vi "Main MSP.vi"() -> ()   [LabVIEW 2025]
uses:
  Support/Move motor.ctl
  Libraries/Control de MaP/Public/Controls/Command to motor.ctl
  Support/Stop motor.ctl
  Support/Home button.ctl
  Support/Program data--cluster.ctl
  Support/Example States.ctl
  Support/Channel configuration--cluster.ctl
  <vilib>/Instr/_visa.llb/VISA Flush IO Buffer Mask.ctl
  Libraries/Control de MaP/Public/Controls/Com Port Options.ctl
  Libraries/TDS1002 Oscilloscope/Trigger config--cluster.ctl
  Libraries/Control de MaP/Public/Write--move.vi
  <vilib>/Waveform/WDTOps.llb/WDT Get XY Value DBL.vi
  Libraries/NI DAQ/NI DAQ.lvlib
  Libraries/TDS1002 Oscilloscope/TDS1002 Oscilloscope.lvlib
  Libraries/Control de MaP/Control de MaP.lvlib
  <resource>/objmgr/daqmx.rc
panel:
  out "Driver listo":bool
  out "DAQ Mod ready":bool
  out "Osc Mod ready":bool
  in  "Connect":bool
  out "Home?":bool
  in  "Home":T1
  out "# mediciones":i32
  in  "Pasos por medición":u16=200
  out "DAQ lista":bool
  out "Osciloscopio listo":bool
  out "Status DAQ":string
  out "Osc":dbl
  in  "Detener motor":T2
  out "End":bool
  out "Posición":dbl format="%.4f"
  in  "Get position":bool
  out "Comando \nenviado":string
  in  "Motor params":T3={"Tipo"=1, "Dirección"=1, "N°. Pasos"=2000, "Frecuencia (Hz)"=255, "Tipo de paso"=2} caption="Parámetros del motor" {"Tipo de paso" items=["", "Medio paso", "Paso completo"]; "Dirección" items=["", "Izquierda", "Derecha"]; "Tipo" items=["", "Unipolar", "Bipolar"]}
  out "XY Graph":cluster{"X":dbl, "Y":dbl}[](graph)
  in  "Mover motor":T4
  in  "Driver de motor":refnum<visa-resource-name>
  in  "Osciloscopio":refnum<visa-resource-name>
  in  "DAQ":u16(ring) items=["Dev3"]
  in  "stop":bool
  # "200 pasos = 0.5mm\n1 paso = 0.0025mm\nCarrera  ~= 40mm"
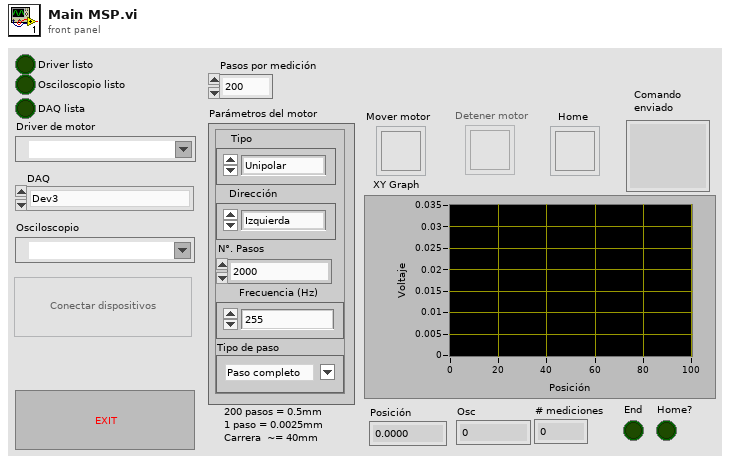
[diagram p1: front panel]
types:
  T1 = typedef "Home button.ctl" = bool
  T2 = typedef "Stop motor.ctl" = bool
  T3 = typedef "Control de MaP.lvlib/Command to motor.ctl" = cluster{"Tipo":u8, "Dirección":u8, "N°. Pasos":u16, "Frecuencia (Hz)":u8, "Tipo de paso":u8}
  T4 = typedef "Move motor.ctl" = bool
  T5 = typedef "Program data--cluster.ctl" = cluster{"Driver de motor":refnum<visa-resource-name>, "DAQ ID":i32, "TDS ID":i32, "Position":dbl, "Moving?":bool, "Pasos por medición":u16, "Motor params":T3}
  T6 = typedef "TDS1002 Oscilloscope.lvlib/Broadcast Events--cluster.ctl" = cluster{"Module Did Init":refnum<user-event>, "Status Updated":refnum<user-event>, "Error Reported":refnum<user-event>, "Module Did Stop":refnum<user-event>, "Update Module Execution Status":refnum<user-event>, "Helper Loop Status Updated":refnum<user-event>, "Device connected":refnum<user-event>, "Device disconnected":refnum<user-event>, "Data acquired":refnum<user-event>, "Configuration applied":refnum<user-event>}
  T7 = typedef "NI DAQ.lvlib/Broadcast Events--cluster.ctl" = cluster{"Module Did Init":refnum<user-event>, "Status Updated":refnum<user-event>, "Error Reported":refnum<user-event>, "Module Did Stop":refnum<user-event>, "Update Module Execution Status":refnum<user-event>, "Digital data acquired":refnum<user-event>, "Device connected":refnum<user-event>, "Connection failed":refnum<user-event>, "Analog data acquired":refnum<user-event>, "Tasks started":refnum<user-event>}
  T8 = typedef "Example States.ctl" = enum16{"Wait", "Validate connection", "Validate modules", "Connect", "Initialize", "Stop motor", "Error", "Exit"}
  T9 = enum8{"Enabled", "Disabled", "Disabled and Grayed Out"}
  T10 = typedef "TDS1002 Oscilloscope.lvlib/Trigger config--cluster.ctl" = cluster{"Trigger Source":i32, "Trigger Mode":i32, "Trigger Slope":i32, "Trigger Coupling":i32, "Trigger Level":dbl}
  T11 = enum16{"All", "DO task", "DI task", "AO task", "AI task"}
  T12 = typedef "TDS1002 Oscilloscope.lvlib/Channel configuration--cluster.ctl" = cluster{"Acquisition Type":i32, "Averaged Waveforms":i32, "Channel":i32, "Probe Attenuation":i32, "Timebase":dbl}
  T13 = typedef "VISA Flush IO Buffer Mask.ctl" = u16
  T14 = typedef "Control de MaP.lvlib/Com Port Options.ctl" = cluster{"baud rate (9600)":u32, "data bits (8)":u16, "parity (0:none)":enum16{"None", "Odd", "Even", "Mark", "Space"}}
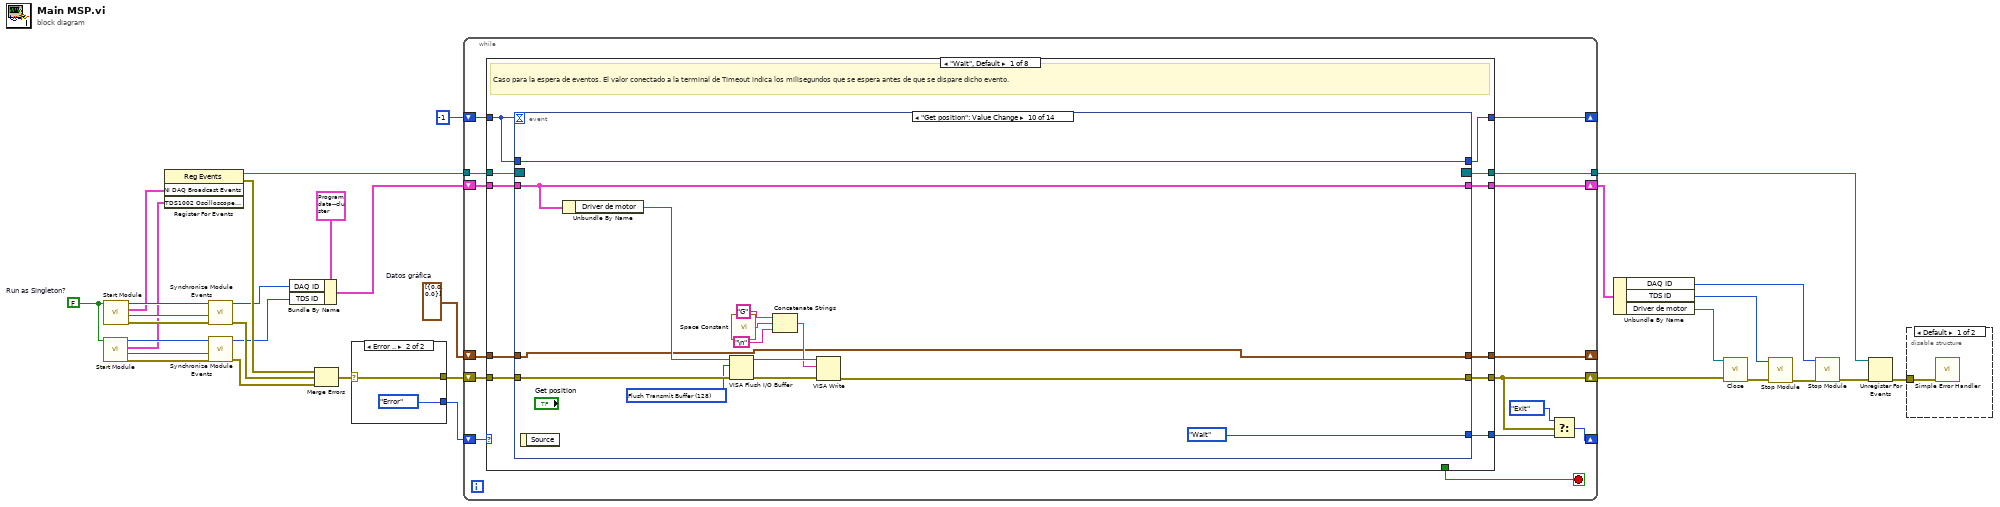
[diagram p0: block diagram]
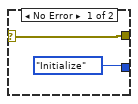
[diagram p2: hidden frame]
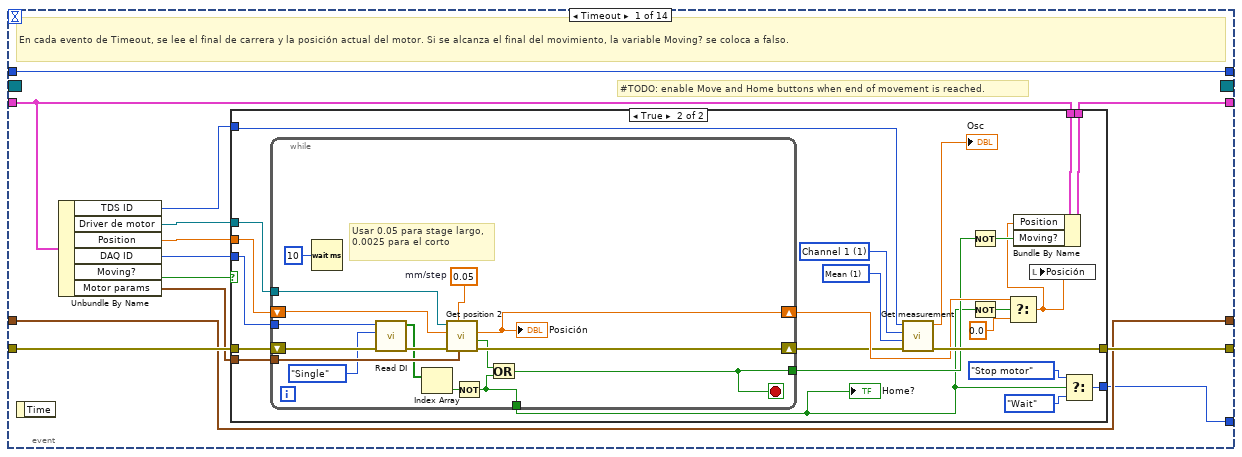
[diagram p3: hidden frame]
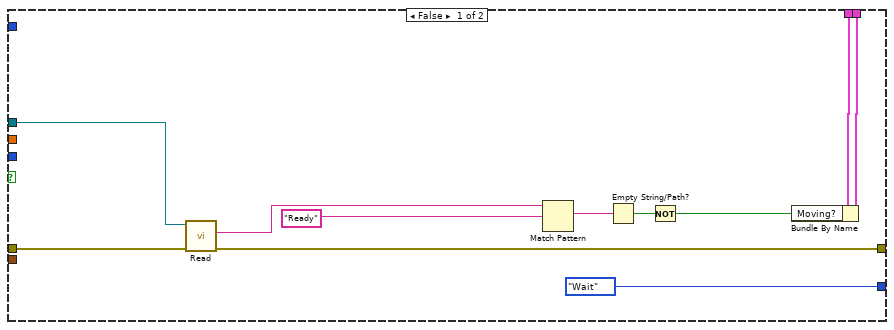
[diagram p4: hidden frame]
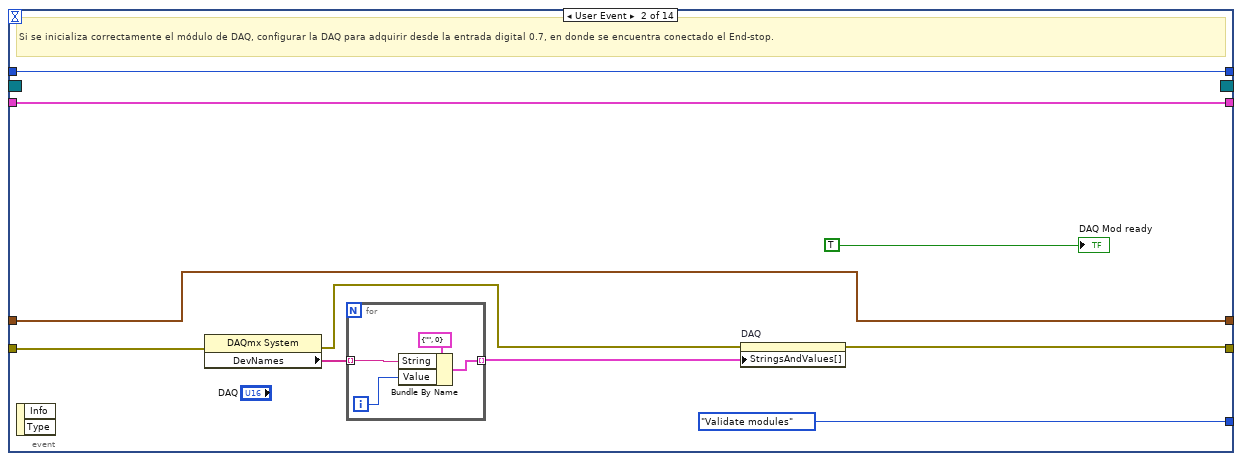
[diagram p5: hidden frame]
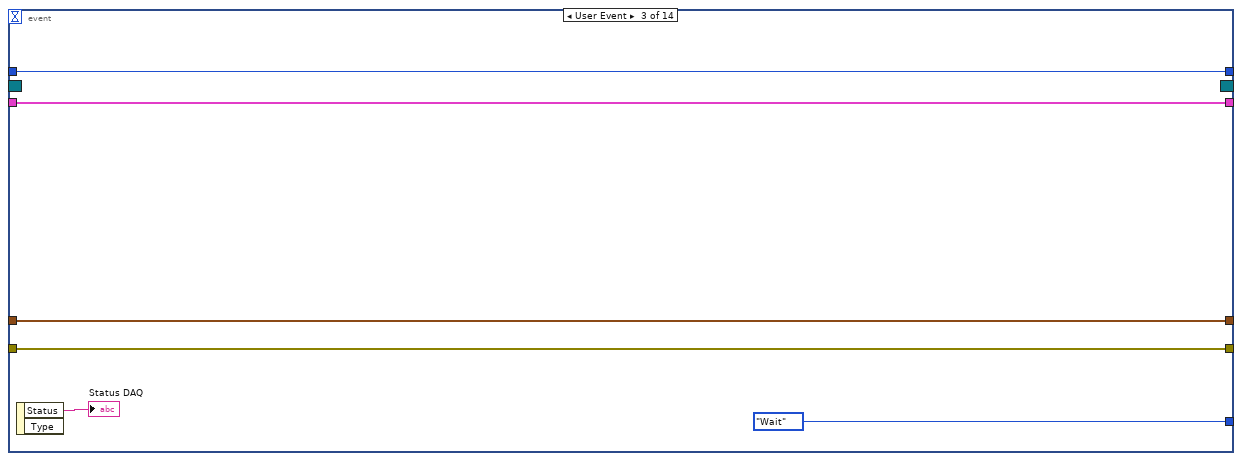
[diagram p6: hidden frame]
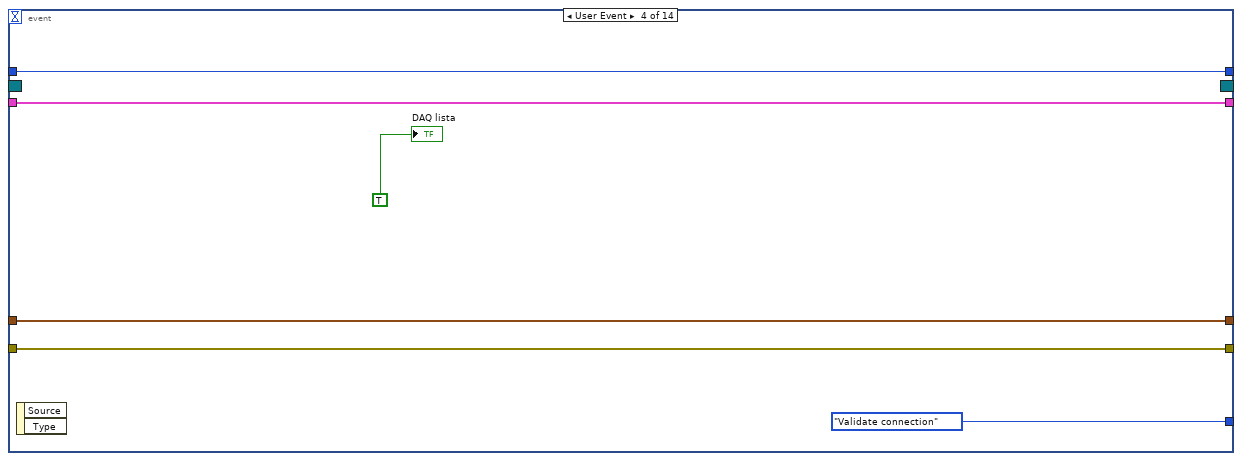
[diagram p7: hidden frame]
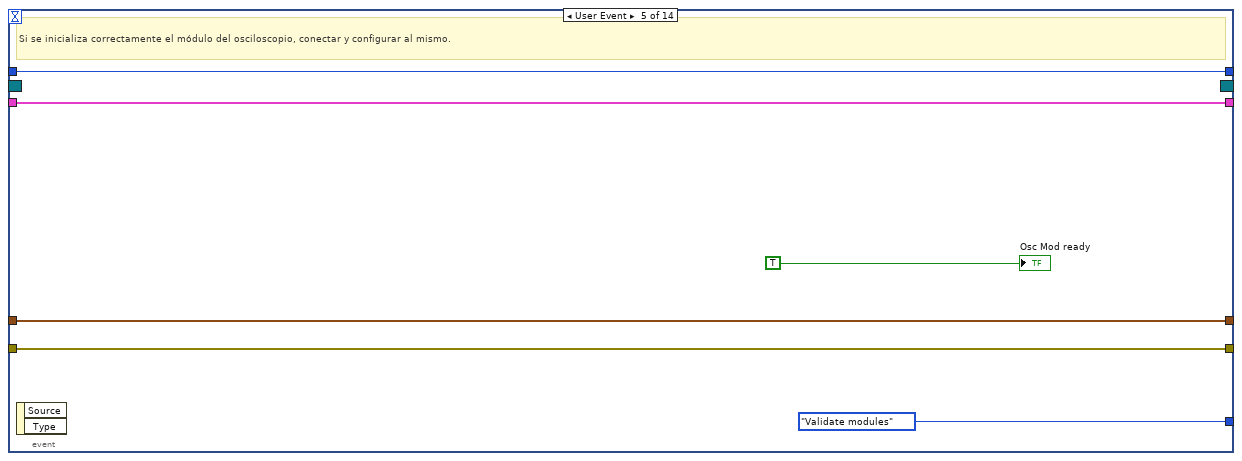
[diagram p8: hidden frame]
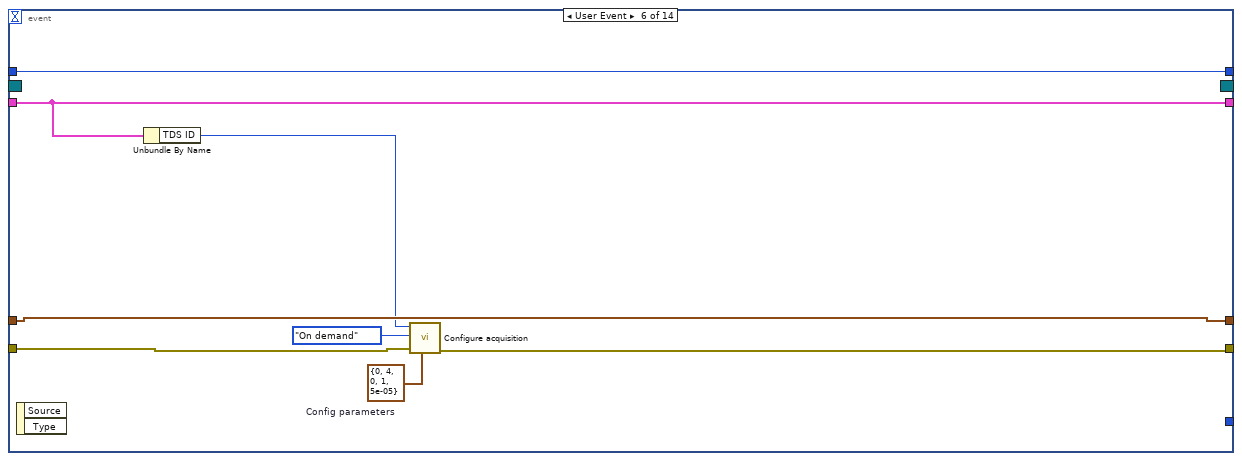
[diagram p9: hidden frame]
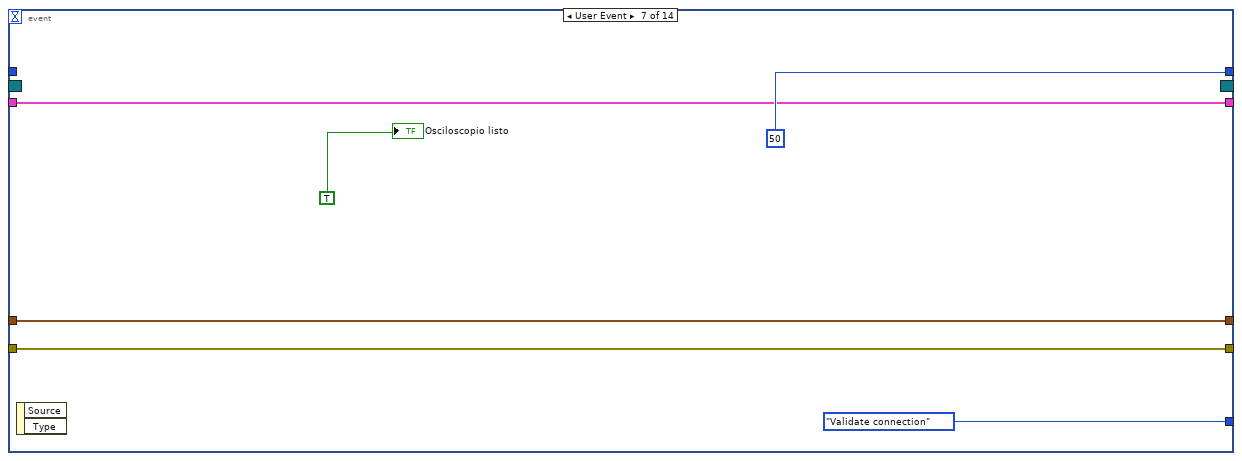
[diagram p10: hidden frame]
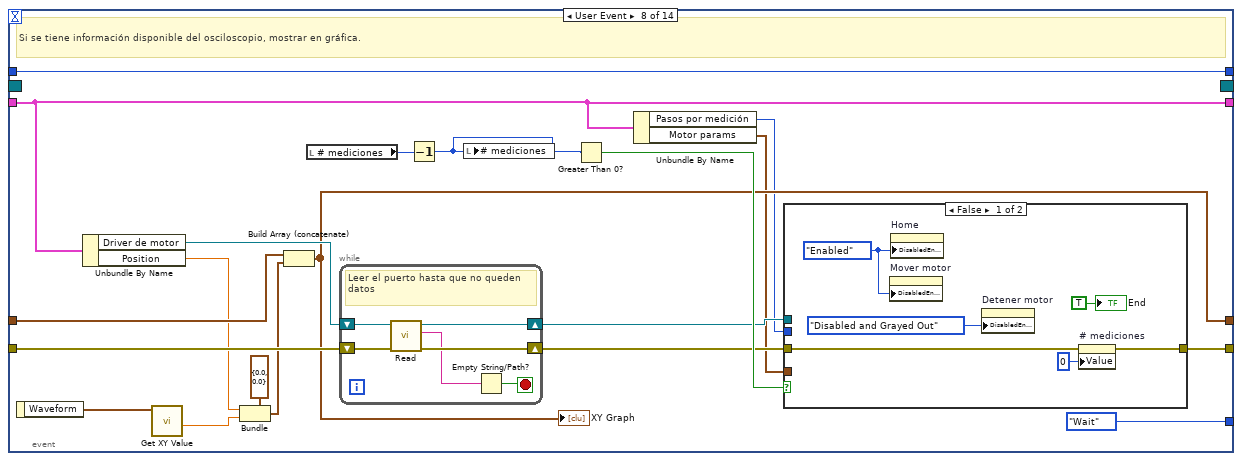
[diagram p11: hidden frame]
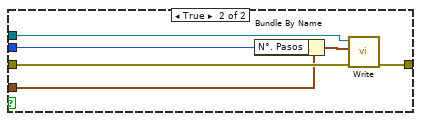
[diagram p12: hidden frame]
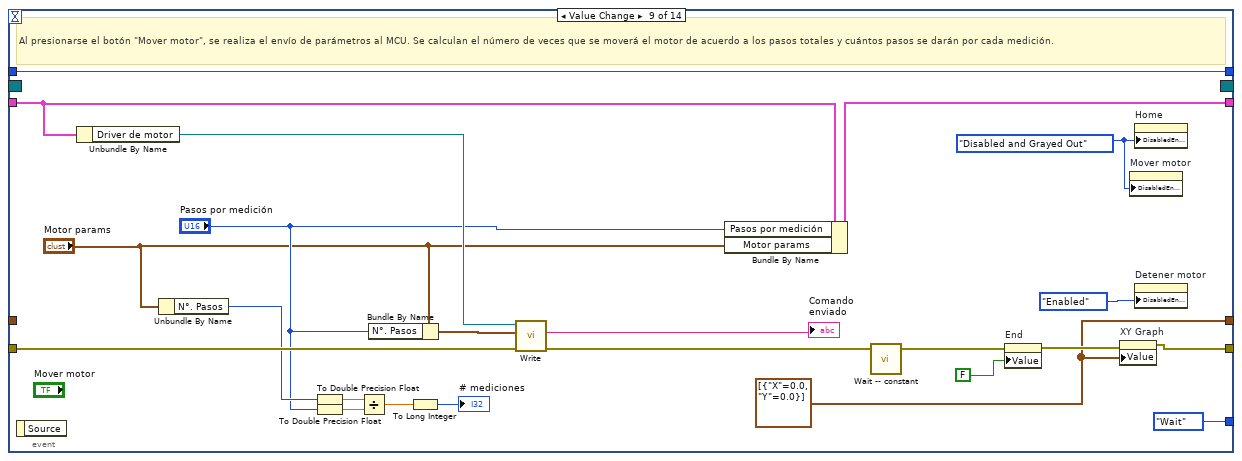
[diagram p13: hidden frame]
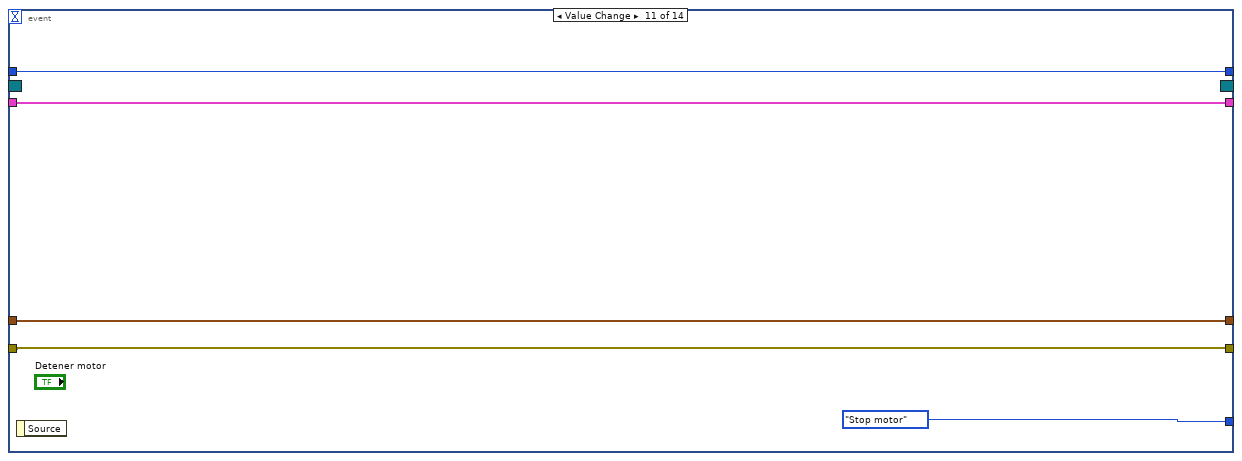
[diagram p14: hidden frame]
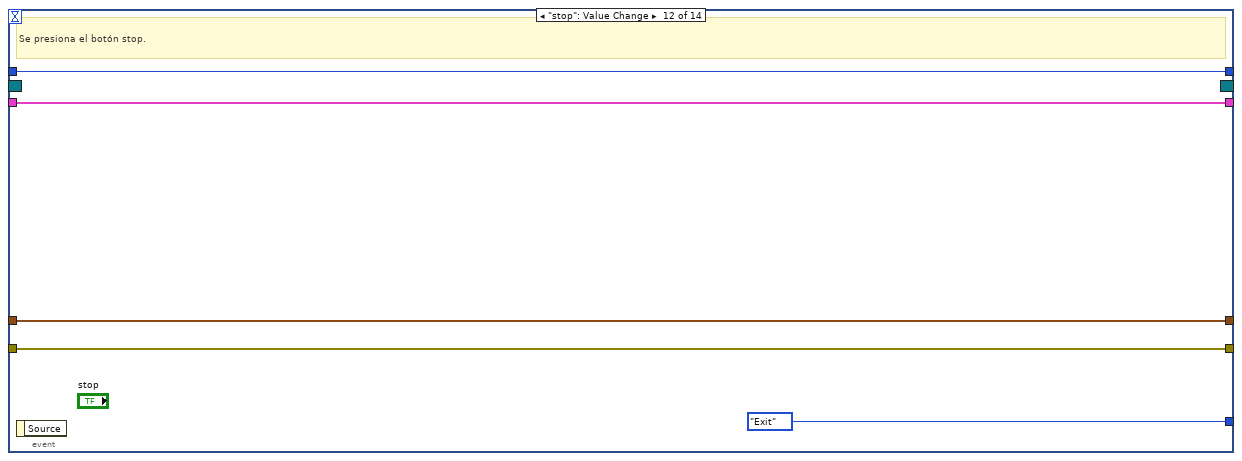
[diagram p15: hidden frame]
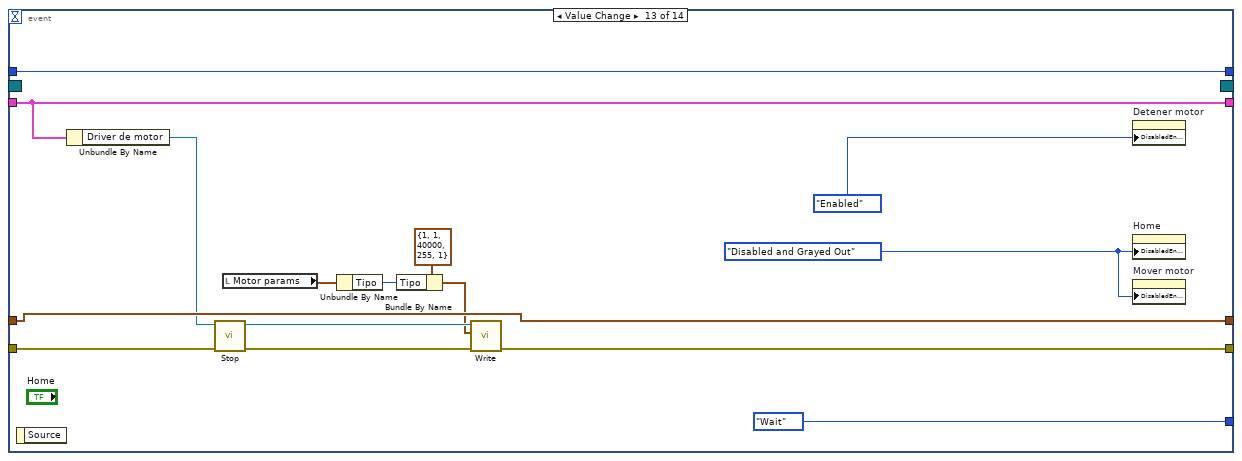
[diagram p16: hidden frame]
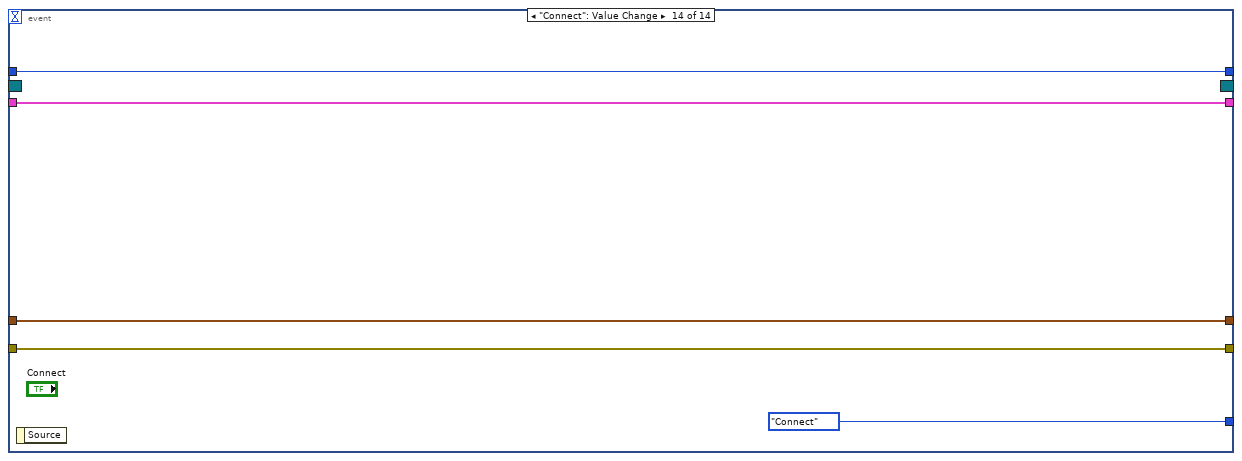
[diagram p17: hidden frame]
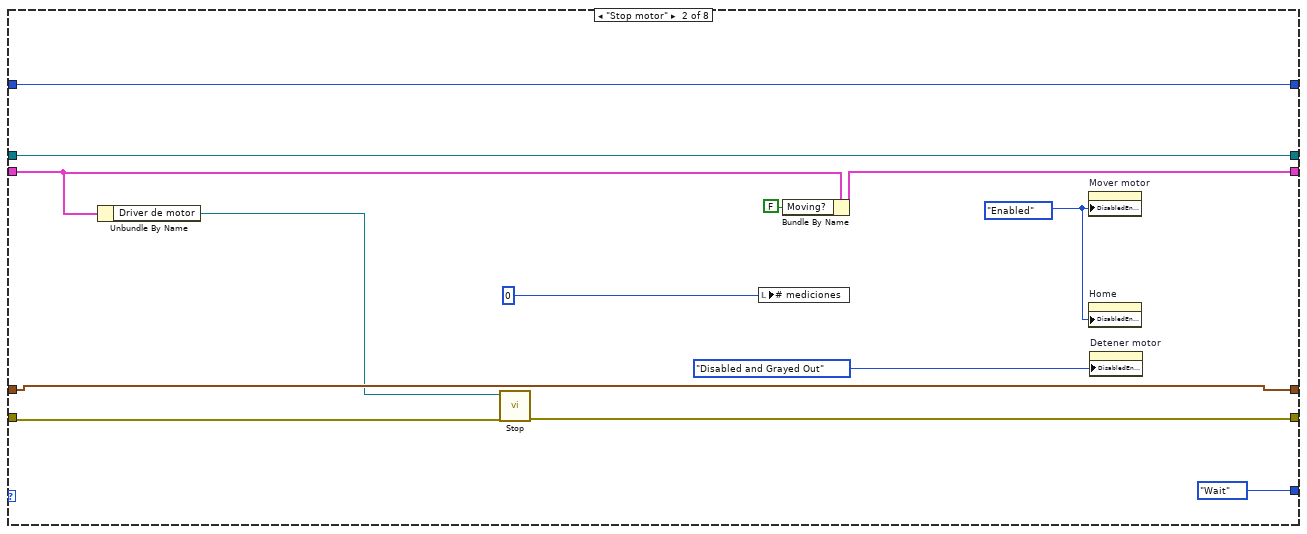
[diagram p18: hidden frame]
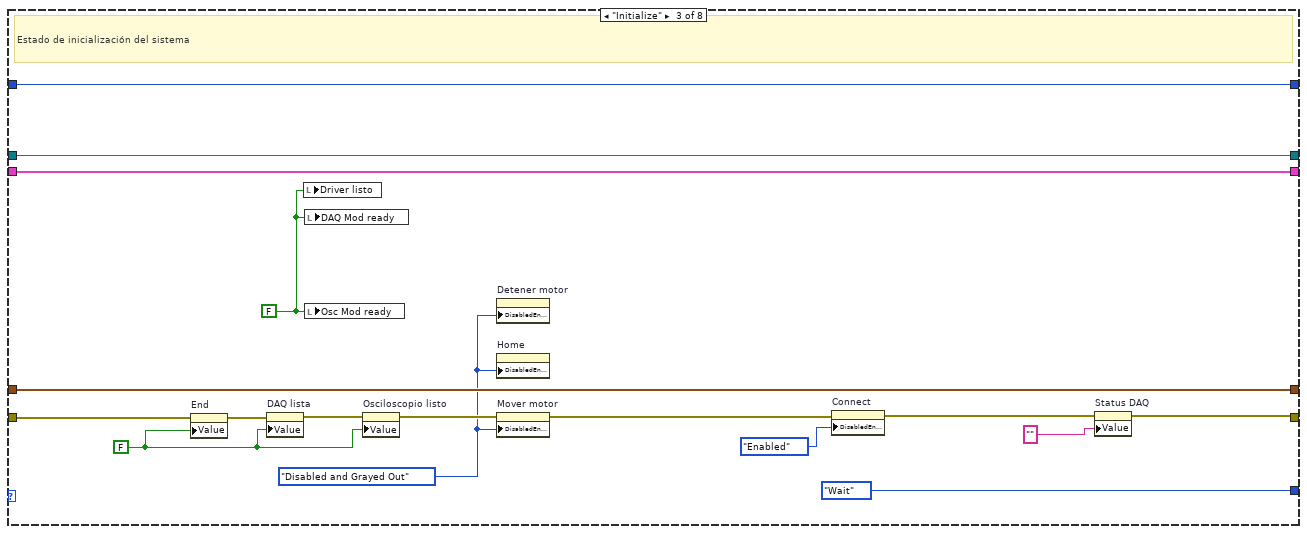
[diagram p19: hidden frame]
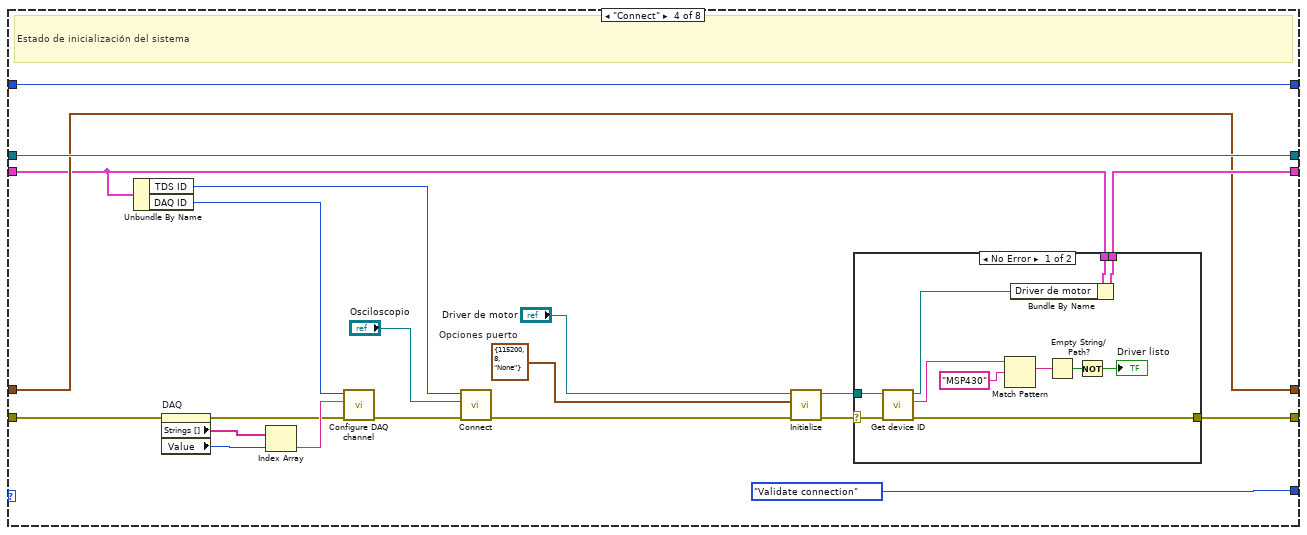
[diagram p20: hidden frame]
diagram:
  w1 = cluster{"X":dbl, "Y":dbl}[] [{"X"=0.0, "Y"=0.0}]  # Datos gráfica
  w21 = FALSE  # Run as Singleton?
  n1 = call "Start Module.vi"("Run as Singleton? (F)"=w21) -> ("error out"=w29:errorcluster, "Wait for Event Sync?"=w27:bool, "TDS1002 Oscilloscope Broadcast Events"=w25:T6, "Module ID"=w28:i32)  [unwired: 7 in]
  n2 = call "Start Module.vi"("Run as Singleton? (F)"=w21) -> ("error out"=w32:errorcluster, "Wait for Event Sync?"=w30:bool, "NI DAQ Broadcast Events"=w26:T7, "Module ID"=w31:i32)  [unwired: 7 in]
  n3 = register-events(w26, w25) -> (reference out=w19:refnum<event-registration>, error out=w22:errorcluster)  [unwired: 2 in]
  n4 = call "Synchronize Module Events.vi"("error in"=w32, "Wait for Event Sync?"=w30, "Module ID in"=w31) -> ("error out"=w23:errorcluster, "Module ID out"=w14:i32)  [unwired: 7 in]
  n5 = call "Synchronize Module Events.vi"("error in"=w29, "Wait for Event Sync?"=w27, "Module ID in"=w28) -> ("error out"=w24:errorcluster, "Module ID out"=w13:i32)  [unwired: 7 in]
  n6 = Bundle By Name(cluster=T5 {"Driver de motor"="", "DAQ ID"=0, "TDS ID"=0, "Position"=0.0, "Moving?"=FALSE, "Pasos por medición"=200, "Motor params"={"Tipo"=1, "Dirección"=1, "N°. Pasos"=2000, "Frecuencia (Hz)"=255, "Tipo de paso"=2}} ("Data"), "DAQ ID"=w14, "TDS ID"=w13) -> (w12:T5)
  n7 = Merge Errors(w22, w23, w24) -> (w5:errorcluster)
  n8 = case shown="Error .." w5 {
    selector: w5 -> [w34 w35]
    tunnel: [w34 w35] -> w4
    tunnel: [Example_States."Initialize" Example_States."Error"] -> w3
    frame No Error {
    }
    frame Error {
    }
  }
  n9 = while {
    shift-right: [w43] -> _
    shift-left: w3 -> [w49]
    tunnel: w19 -> [w48]
    tunnel: [w47] -> w17
    shift-right: [w46] -> w11
    shift-left: w12 -> [w45]
    shift-right: [w42] -> w9
    shift-left: w4 -> [w51]
    shift-right: [w38] -> _
    shift-left: w1 -> [w39]
    shift-right: [w37] -> _
    shift-left: -1 -> [w40]
    stop <- w50 stop-if-true
    n10 = case shown="\"Wait\", Default" w49 {
      tunnel: w51 -> [w62 w286 w302 w317 w346 w362 w386 w402]
      tunnel: [w61 w280 w297 w308 w345 w363 w383 w401] -> w42
      tunnel: [_ _ _ _ _ _ w397 _] -> w50
      tunnel: [w60 Example_States."Wait" ("Not used") Example_States."Wait" ("Not used") Example_States."Validate connection" ("Not used") Example_States."Wait" ("Not used") Example_States."Wait" ("Not used") w394 Example_States."Exit" ("Not used")] -> w44
      tunnel: w48 -> [w59 w281 w305 w326 w354 w369 w398 w405]
      tunnel: [w58 w281 w305 w326 w354 w369 w398 w405] -> w47
      tunnel: [w56 w282 w295 w324 w353 w360 w393 w404] -> w46
      tunnel: w45 -> [w57 w283 w295 w316 w353 w360 w393 w404]
      tunnel: w40 -> [w53 w289 w298 w322 w351 w367 w384 w399]
      tunnel: w39 -> [w55 w285 w299 w323 w352 w368 w385 w400]
      tunnel: [w54 w285 w299 w323 w352 w368 w385 w400] -> w38
      tunnel: [w52 w289 w298 w322 w351 w367 w384 w399] -> w37
      frame "Wait", Default {
        # "Caso para la espera de eventos. El valor conectado a la terminal de Timeout indica los milisegundos que se espera antes de que se dispare dicho evento."
        n11 = event shown="[9] \"Get position\": Value Change" {
          selector: w59 -> [_ _ _ _ _ _ _ _ _ _ _ _ _ _]
          dyn-events: [_ _ _ _ _ _ _ _ _ _ _ _ _ _] -> w58
          timeout: w53 -> [_ _ _ _ _ _ _ _ _ _ _ _ _ _]
          tunnel: w62 -> [w67 w129 w143 w150 w153 w162 w171 w184 w231 w244 w249 w256 w269 w272]
          tunnel: [w75 w128 w143 w150 w153 w158 w171 w190 w218 w246 w249 w256 w265 w272] -> w61
          tunnel: [w63 Example_States."Validate modules" Example_States."Wait" Example_States."Validate connection" Example_States."Validate modules" _ Example_States."Validate connection" Example_States."Wait" Example_States."Wait" Example_States."Wait" Example_States."Stop motor" Example_States."Exit" Example_States."Wait" Example_States."Connect"] -> w60
          tunnel: w57 -> [w74 w135 w145 w151 w156 w161 w166 w175 w216 w245 w248 w254 w268 w276]
          tunnel: [w73 w135 w145 w151 w156 w161 w166 w175 w212 w245 w248 w254 w268 w276] -> w56
          tunnel: w55 -> [w66 w133 w142 w148 w155 w165 w168 w181 _ w234 w247 w253 w271 w275]
          tunnel: [w66 w133 w142 w148 w155 w165 w168 w176 w217 w234 w247 w253 w271 w275] -> w54
          tunnel: w53 -> [w64 w132 w140 w147 w154 w164 _ w172 w213 w233 w250 w252 w263 w274]
          tunnel: [w64 w132 w140 w147 w154 w164 50 w172 w213 w233 w250 w252 w263 w274] -> w52
          event Timeout {
            # "#TODO: enable Move and Home buttons when end of movement is reached."
            # "En cada evento de Timeout, se lee el final de carrera y la posición actual del motor. Si se alcanza el final del movimiento, la variable Moving? se coloca a falso."
            n12 = event-data() -> ()  [unwired: 1 in, 1 out]
            n13 = Unbundle By Name(w74) -> ("TDS ID"=w68:i32, "Driver de motor"=w70:refnum<visa-resource-name>, "Position"=w71:dbl, "DAQ ID"=w72:i32, "Moving?"=w69:bool, "Motor params"=w65:T3)
            n14 = case shown="True" w69 {
              tunnel: w70 -> [w85 w105]
              tunnel: [w86 w100] -> w75
              tunnel: w74 -> [w84 w109]
              tunnel: [w80 w108] -> w73
              tunnel: w72 -> [_ w98]
              tunnel: w71 -> [_ w103]
              tunnel: w68 -> [_ w89]
              tunnel: w67 -> [w77 w101]
              tunnel: w65 -> [_ w99]
              tunnel: [Example_States."Wait" ("Not used") w96] -> w63
              frame False {
                n15 = call "Read.vi"("error in (no error)"=w77, "VISA resource name"=w85) -> ("error out"=w86:errorcluster, "Recibo de Datos"=w83:string)  [unwired: 6 in, 2 out]
                n16 = Match Pattern(string=w83, regular expression="Ready") -> (match substring=w81:string)  [unwired: 1 in, 3 out]
                n17 = Empty String/Path?(string/path=w81) -> (empty?=w79:bool)
                n18 = Not(x=w79) -> (.not. x?=w78:bool)
                n19 = Bundle By Name(cluster=w84, "Moving?"=w78) -> (w80:T5)
              }
              frame True {
                w106 = 1 items=["Frequency", "Mean", "Period", "Pulse Duty", "Peak to Peak", "Cycle RMS", "Minimum", "Maximum", "Rise Time", "Fall Time", "Positive Width", "Negative Width", "Amplitude", "Cycle Mean", "High", "Low", "Negative Duty", "Positive Overshoot", "Negative Overshoot", "Cursor Mean", "Burst Width", "Positive Pulse Count", "Negative Pulse Count", "Rising Edge Count", "Falling Edge Count", "Area", "Cycle Area", "RMS", "Cursor RMS"] ("Measurement Type")
                w107 = 1 items=["Channel 1"=1, "Channel 2"=2, "Channel 3"=3, "Channel 4"=4] ("Channel")
                n20 = while {
                  tunnel: w105 -> [w124]
                  shift-right: [w121] -> w92
                  shift-left: w103 -> [w123]
                  shift-right: [w125] -> w90
                  shift-left: w101 -> [w118]
                  tunnel: [w113] -> w88
                  tunnel: w99 -> [w119]
                  tunnel: w98 -> [w116]
                  tunnel: [w111] -> w87
                  stop <- w113 stop-if-true
                  w122 = 0.05  # mm/step
                  # "Usar 0.05 para stage largo, 0.0025 para el corto"
                  n21 = Wait (ms)(milliseconds to wait=u32 10) -> ()  [unwired: 1 out]
                  n22 = call "Read DI.vi"("error in"=w118, "Samples"=enum16{"Single", "Multiple"}."Single", "Module ID"=w116) -> ("error out"=w117:errorcluster, "Data"=w114:bool[])  [unwired: 6 in, 1 out]
                  n23 = Index Array(array=w114) -> (element=w112:bool)  [unwired: 1 in]
                  n24 = call "Get position 2.vi"("Motor params"=w119, "mm/step"=w122, "error in (no error)"=w117, "Position in"=w123, "VISA resource name in"=w124) -> ("error out"=w125:errorcluster, "End?"=w110:bool, "Positions out"=w121:dbl)  [unwired: 3 in, 1 out]
                  "Posición" <- w121
                  n25 = Not(x=w112) -> (.not. x?=w111:bool)
                  n26 = Or(x=w110, y=w111) -> (x .or. y?=w113:bool)
                }
                "Home?" <- w87
                n27 = call "Get measurement.vi"("error in"=w90, "Measurement Type"=w106, "Channel"=w107, "Module ID"=w89) -> ("error out"=w100:errorcluster, "Value"=→"Osc":dbl)  [unwired: 5 in, 1 out]
                n28 = Not(x=w88) -> (.not. x?=w102:bool)
                n29 = Not(x=w87) -> (.not. x?=w93:bool)
                n30 = Select(t=w92, s=w93, f=0.0) -> (s? t:f=w91:dbl)
                n31 = Bundle By Name(cluster=w109, "Position"=w91, "Moving?"=w102) -> (w108:T5)
                n32 = local write "Posición"(w91) -> ()
                n33 = Select(t=Example_States."Stop motor", s=w87, f=Example_States."Wait" ("Not used")) -> (s? t:f=w96:T8)
              }
            }
          }
          event User Event {
            # "Si se inicializa correctamente el módulo de DAQ, configurar la DAQ para adquirir desde la entrada digital 0.7, en donde se encuentra conectado el End-stop."
            n34 = event-data() -> ()  [unwired: 1 in, 2 out]
            n35 = property class="DAQmx System"(error in=w129) -> (error out=w131:errorcluster, "DevNames"=w130:tag[])  [unwired: 1 in, 1 out]
            n36 = for {
              tunnel: w130 -> [w136] mode=indexing
              tunnel: [w137] -> w127 mode=indexing
              i -> [w138]
              n37 = Bundle By Name(cluster=cluster{"String":string, "Value":u16} {"String"="", "Value"=0} ("Cluster"), "String"=w136, "Value"=w138) -> (w137:cluster{"String":string, "Value":u16})
            }
            n38 = property on="DAQ" class="Ring (strict)"(error in=w131, "StringsAndValues[]"=w127) -> (error out=w128:errorcluster)  [unwired: 1 in, 1 out]
            "DAQ Mod ready" <- TRUE ("DAQ Mod ready")
          }
          event User Event {
            n39 = event-data() -> ("Status"=→"Status DAQ":string)  [unwired: 1 in, 1 out]
          }
          event User Event {
            n40 = event-data() -> ()  [unwired: 1 in, 2 out]
            "DAQ lista" <- TRUE ("DAQ lista")
          }
          event User Event {
            # "Si se inicializa correctamente el módulo del osciloscopio, conectar y configurar al mismo."
            n41 = event-data() -> ()  [unwired: 1 in, 2 out]
            "Osc Mod ready" <- TRUE ("Ocs Mod ready")
          }
          event User Event {
            w163 = T12 {"Acquisition Type"=0, "Averaged Waveforms"=4, "Channel"=0, "Probe Attenuation"=1, "Timebase"=5e-05}  # Config parameters
            n42 = event-data() -> ()  [unwired: 1 in, 2 out]
            n43 = Unbundle By Name(w161) -> ("TDS ID"=w160:i32)
            n44 = call "Configure acquisition.vi"("Config parameters"=w163, "error in"=w162, "Type"=enum16{"On demand", "Continous"}."On demand", "Module ID"=w160) -> ("error out"=w158:errorcluster)  [unwired: 7 in]
          }
          event User Event {
            n45 = event-data() -> ()  [unwired: 1 in, 2 out]
            "Osciloscopio listo" <- TRUE
          }
          event User Event {
            # "Si se tiene información disponible del osciloscopio, mostrar en gráfica."
            n46 = event-data() -> ("Waveform"=w182:waveform(dbl))  [unwired: 1 in]
            n47 = Unbundle By Name(w175) -> ("Driver de motor"=w186:refnum<visa-resource-name>, "Position"=w178:dbl)
            n48 = call-poly <vilib>:"Get XY Value.vi"("waveform in"=w182) -> ("Y value"=w179:dbl)  [unwired: 6 in, 4 out]
            n49 = Bundle(cluster=cluster{"X":dbl, "Y":dbl} {"X"=0.0, "Y"=0.0}, "X"=w178, "Y"=w179) -> (w177:cluster{"X":dbl, "Y":dbl})
            n50 = Build Array (concatenate)(w181, w177) -> (w176:cluster{"X":dbl, "Y":dbl}[])
            "XY Graph" <- w176
            n51 = local read "# mediciones"() -> (w189:i32)
            n52 = while {
              shift-right: [w196] -> w185
              shift-left: w186 -> [w197]
              shift-right: [w194] -> w183
              shift-left: w184 -> [w195]
              stop <- w193 stop-if-true
              # "Leer el puerto hasta que no queden datos"
              n53 = call "Read.vi"("error in (no error)"=w195, "VISA resource name"=w197) -> ("error out"=w194:errorcluster, "Recibo de Datos"=w192:string, "VISA resource name out"=w196:refnum<visa-resource-name>)  [unwired: 6 in, 1 out]
              n54 = Empty String/Path?(string/path=w192) -> (empty?=w193:bool)
            }
            n55 = Decrement(x=w189) -> (x-1=w188:i32)
            n56 = local write "# mediciones"(w188) -> ()
            n57 = Greater Than 0?(x=w188) -> (x > 0?=w187:bool)
            n58 = Unbundle By Name(w175) -> ("Pasos por medición"=w174:u16, "Motor params"=w173:T3)
            n59 = case shown="False" w187 {
              tunnel: w183 -> [w202 w208]
              tunnel: [w201 w207] -> w190
              tunnel: w185 -> [_ w206]
              tunnel: w174 -> [_ w205]
              tunnel: w173 -> [_ w204]
              frame False {
                w198 = T9."Enabled" ("Disabled")
                n60 = property on="Mover motor" class="Bool"("DisabledEnum"=w198) -> ()  [unwired: 2 in, 2 out]
                n61 = property on="Home" class="Bool"("DisabledEnum"=w198) -> ()  [unwired: 2 in, 2 out]
                n62 = property on="Detener motor" class="Bool"("DisabledEnum"=T9."Disabled and Grayed Out" ("Disabled")) -> ()  [unwired: 2 in, 2 out]
                n63 = property on="# mediciones" class="DigNum (strict)"(error in=w202, "Value"=0 ("# mediciones")) -> (error out=w201:errorcluster)  [unwired: 1 in, 1 out]
                "End" <- TRUE ("End")
              }
              frame True {
                n64 = Bundle By Name(cluster=w204, "N°. Pasos"=w205) -> (w209:T3)
                n65 = call-poly "Write.vi"("error in (no error)"=w208, "Comando"=w209, "VISA resource name"=w206) -> ("error out"=w207:errorcluster)  [unwired: 6 in, 2 out]
              }
            }
          }
          event Value Change {
            w210 = T9."Disabled and Grayed Out" ("Disabled")
            w217 = cluster{"X":dbl, "Y":dbl}[] [{"X"=0.0, "Y"=0.0}] ("XY Graph")
            # "Al presionarse el botón \"Mover motor\", se realiza el envío de parámetros al MCU. Se calculan el número de veces que se moverá el motor de acuerdo a los pasos totales y cuántos pasos se darán por cada medición."
            n66 = event-data() -> ()  [unwired: 1 in, 1 out]
            n67 = Unbundle By Name(w216) -> ("Driver de motor"=w230:refnum<visa-resource-name>)
            n68 = Unbundle By Name("Motor params") -> ("N°. Pasos"=w229:u16)
            n69 = To Double Precision Float(number=w229) -> (double precision float=w228:dbl)
            n70 = To Double Precision Float(number="Pasos por medición") -> (double precision float=w223:dbl)
            n71 = Divide(x=w228, y=w223) -> (x/y=w227:dbl)
            n72 = Bundle By Name(cluster="Motor params", "N°. Pasos"="Pasos por medición") -> (w225:T3)
            n73 = To Long Integer(number=w227) -> (32bit integer=→"# mediciones":i32)
            n74 = call-poly "Write.vi"("error in (no error)"=w231, "Comando"=w225, "VISA resource name"=w230) -> ("error out"=w221:errorcluster, "Comando(string)"=→"Comando \nenviado":string)  [unwired: 6 in, 1 out]
            n75 = Bundle By Name(cluster=w216, "Pasos por medición"="Pasos por medición", "Motor params"="Motor params") -> (w212:T5)
            n76 = call "Wait -- constant.vi"("error in (no error)"=w221) -> ("error out"=w220:errorcluster)  [unwired: 6 in]
            n77 = property on="End" class="Bool (strict)"(error in=w220, "Value"=FALSE ("End")) -> (error out=w219:errorcluster)  [unwired: 1 in, 1 out]
            n78 = property on="XY Graph" class="XYGraph (strict)"(error in=w219, "Value"=w217) -> (error out=w218:errorcluster)  [unwired: 1 in, 1 out]
            n79 = property on="Mover motor" class="Bool"("DisabledEnum"=w210) -> ()  [unwired: 2 in, 2 out]
            n80 = property on="Home" class="Bool"("DisabledEnum"=w210) -> ()  [unwired: 2 in, 2 out]
            n81 = property on="Detener motor" class="Bool"("DisabledEnum"=T9."Enabled" ("Disabled")) -> ()  [unwired: 2 in, 2 out]
          }
          event "Get position": Value Change {
            w240 = T13 128 items=["Flush Receive Buffer"=16, "Write Transmit Buffer to Device"=32, "Flush Receive Buffer (No I/O)"=64, "Flush Transmit Buffer"=128] ("Mask")
            n82 = event-data() -> ()  [unwired: 1 in, 1 out]
            n83 = Unbundle By Name(w245) -> ("Driver de motor"=w242:refnum<visa-resource-name>)
            n84 = VISA Flush I/O Buffer(VISA resource name=w242, mask (16)=w240, error in (no error)=w244) -> (VISA resource name out=w241:refnum<visa-resource-name>, error out=w243:errorcluster)
            n85 = call <vilib>:"Space Constant.vi"() -> ("String"=w236:string)
            n86 = Concatenate Strings("G" ("write buffer"), w236, "\n") -> (w238:string)
            n87 = VISA Write(VISA resource name=w241, write buffer=w238, error in (no error)=w243) -> (error out=w246:errorcluster)  [unwired: 2 out]
          }
          event Value Change {
            n88 = event-data() -> ()  [unwired: 1 in, 1 out]
          }
          event "stop": Value Change {
            # "Se presiona el botón stop."
            n89 = event-data() -> ()  [unwired: 1 in, 1 out]
          }
          event Value Change {
            w257 = T9."Disabled and Grayed Out" ("Disabled")
            n90 = event-data() -> ()  [unwired: 1 in, 1 out]
            n91 = Unbundle By Name(w268) -> ("Driver de motor"=w267:refnum<visa-resource-name>)
            n92 = call "Stop.vi"("error in (no error)"=w269, "VISA resource name"=w267) -> ("error out"=w266:errorcluster, "VISA resource name out"=w264:refnum<visa-resource-name>)  [unwired: 8 in]
            n93 = local read "Motor params"() -> (w260:T3)
            n94 = Unbundle By Name(w260) -> ("Tipo"=w259:u8)
            n95 = Bundle By Name(cluster=T3 {"Tipo"=1, "Dirección"=1, "N°. Pasos"=40000, "Frecuencia (Hz)"=255, "Tipo de paso"=1} ("Comando"), "Tipo"=w259) -> (w261:T3)
            n96 = call-poly "Write.vi"("error in (no error)"=w266, "Comando"=w261, "VISA resource name"=w264) -> ("error out"=w265:errorcluster)  [unwired: 6 in, 2 out]
            n97 = property on="Detener motor" class="Bool"("DisabledEnum"=T9."Enabled" ("Disabled")) -> ()  [unwired: 2 in, 2 out]
            n98 = property on="Home" class="Bool"("DisabledEnum"=w257) -> ()  [unwired: 2 in, 2 out]
            n99 = property on="Mover motor" class="Bool"("DisabledEnum"=w257) -> ()  [unwired: 2 in, 2 out]
          }
          event "Connect": Value Change {
            n100 = event-data() -> ()  [unwired: 1 in, 1 out]
          }
        }
      }
      frame "Stop motor" {
        w278 = T9."Enabled" ("Disabled")
        n101 = Unbundle By Name(w283) -> ("Driver de motor"=w284:refnum<visa-resource-name>)
        n102 = call "Stop.vi"("error in (no error)"=w286, "VISA resource name"=w284) -> ("error out"=w280:errorcluster)  [unwired: 8 in, 1 out]
        n103 = local write "# mediciones"(0 ("# mediciones")) -> ()
        n104 = Bundle By Name(cluster=w283, "Moving?"=FALSE) -> (w282:T5)
        n105 = property on="Mover motor" class="Bool"("DisabledEnum"=w278) -> ()  [unwired: 2 in, 2 out]
        n106 = property on="Home" class="Bool"("DisabledEnum"=w278) -> ()  [unwired: 2 in, 2 out]
        n107 = property on="Detener motor" class="Bool"("DisabledEnum"=T9."Disabled and Grayed Out" ("Disabled")) -> ()  [unwired: 2 in, 2 out]
      }
      frame "Initialize" {
        w291 = FALSE ("Ocs Mod ready")
        w300 = FALSE ("DAQ lista")
        w292 = T9."Disabled and Grayed Out" ("Disabled")
        # "Estado de inicialización del sistema"
        n108 = property on="End" class="Bool (strict)"(error in=w302, "Value"=w300) -> (error out=w301:errorcluster)  [unwired: 1 in, 1 out]
        n109 = property on="DAQ lista" class="Bool (strict)"(error in=w301, "Value"=w300) -> (error out=w304:errorcluster)  [unwired: 1 in, 1 out]
        n110 = local write "Driver listo"(w291) -> ()
        n111 = local write "DAQ Mod ready"(w291) -> ()
        n112 = local write "Osc Mod ready"(w291) -> ()
        n113 = property on="Osciloscopio listo" class="Bool (strict)"(error in=w304, "Value"=w300) -> (error out=w303:errorcluster)  [unwired: 1 in, 1 out]
        n114 = property on="Detener motor" class="Bool"("DisabledEnum"=w292) -> ()  [unwired: 2 in, 2 out]
        n115 = property on="Home" class="Bool"("DisabledEnum"=w292) -> ()  [unwired: 2 in, 2 out]
        n116 = property on="Mover motor" class="Bool"(error in=w303, "DisabledEnum"=w292) -> (error out=w294:errorcluster)  [unwired: 1 in, 1 out]
        n117 = property on="Connect" class="Bool"(error in=w294, "DisabledEnum"=T9."Enabled" ("Disabled")) -> (error out=w293:errorcluster)  [unwired: 1 in, 1 out]
        n118 = property on="Status DAQ" class="Str"(error in=w293, "Value"="" ("Status DAQ")) -> (error out=w297:errorcluster)  [unwired: 1 in, 1 out]
      }
      frame "Connect" {
        w325 = T14 {"baud rate (9600)"=115200, "data bits (8)"=8, "parity (0:none)"=enum."None"}  # Opciones puerto
        # "Estado de inicialización del sistema"
        n119 = Unbundle By Name(w316) -> ("TDS ID"=w312:i32, "DAQ ID"=w315:i32)
        n120 = property on="DAQ" class="Ring (strict)"(error in=w317) -> (error out=w320:errorcluster, "Strings []"=w319:string[], "Value"=w318:u16)  [unwired: 1 in, 1 out]
        n121 = Index Array(array=w319, index=w318) -> (element=w321:string)
        n122 = call "Configure DAQ channel.vi"("error in (no error)"=w320, "String"=w321, "DAQ ID"=w315) -> ("error out"=w311:errorcluster)  [unwired: 8 in]
        n123 = call "Connect.vi"("error in"=w311, "VISA resource name"="Osciloscopio", "Module ID"=w312) -> ("error out"=w310:errorcluster)  [unwired: 8 in]
        n124 = call "Initialize.vi"("error in (no error)"=w310, "Opciones puerto"=w325, "Puerto Serial"="Driver de motor") -> ("error out"=w309:errorcluster, "VISA resource name out"=w307:refnum<visa-resource-name>)  [unwired: 7 in]
        n125 = case shown="No Error" w309 {
          selector: w309 -> [w336 w343]
          tunnel: [w338 w344] -> w324
          tunnel: w316 -> [w337 w344]
          tunnel: [w335 w342] -> w308
          tunnel: w307 -> [w334 _]
          frame No Error {
            n126 = call "Get device ID.vi"("error in (no error)"=w336, "VISA resource name in"=w334) -> ("error out"=w335:errorcluster, "ID"=w332:string, "VISA Refnum out"=w333:refnum<visa-resource-name>)  [unwired: 7 in]
            n127 = Match Pattern(string=w332, regular expression="MSP430" ("x")) -> (match substring=w330:string)  [unwired: 1 in, 3 out]
            n128 = Bundle By Name(cluster=w337, "Driver de motor"=w333) -> (w338:T5)
            n129 = Empty String/Path?(string/path=w330) -> (empty?=w329:bool)
            n130 = Not(x=w329) -> (.not. x?=→"Driver listo":bool)
          }
          frame Error {
            w341 = -1073807346  # Driver was not connected.
            n131 = One Button Dialog(message="Driver no conectado.") -> ()  [unwired: 1 in, 1 out]
            n132 = property on="Connect" class="Bool"("DisabledEnum"=T9."Enabled" ("Disabled")) -> ()  [unwired: 2 in, 2 out]
            n133 = call <vilib>:"Clear Errors.vi"("error in (no error)"=w343, "specific error code to clear (0: all)"=w341) -> ("error out"=w342:errorcluster)  [unwired: 4 in, 1 out]
          }
        }
      }
      frame "Validate modules" {
        n134 = local read "DAQ Mod ready"() -> (w350:bool)
        n135 = local read "Osc Mod ready"() -> (w349:bool)
        n136 = And(x=w350, y=w349) -> (x .and. y?=w347:bool)
        n137 = case shown="False" w347 {
          tunnel: w346 -> [w355 w357]
          tunnel: [w355 w356] -> w345
          frame False {
          }
          frame True {
            n138 = property on="Connect" class="Bool"(error in=w357, "DisabledEnum"=T9."Enabled" ("Disabled")) -> (error out=w356:errorcluster)  [unwired: 1 in, 1 out]
          }
        }
      }
      frame "Validate connection" {
        n139 = local read "Osciloscopio listo"() -> (w365:bool)
        n140 = local read "Driver listo"() -> (w359:bool)
        n141 = local read "DAQ lista"() -> (w364:bool)
        n142 = Compound Arithmetic op=AND(w359, w364, w365) -> (w366:bool)
        n143 = case shown="True" w366 {
          tunnel: w362 -> [w370 w378]
          tunnel: [w370 w374] -> w363
          tunnel: w360 -> [_ w373]
          frame False {
          }
          frame True {
            w377 = T9."Enabled" ("Disabled")
            n144 = Unbundle By Name(w373) -> ("TDS ID"=w372:i32)
            n145 = property on="Home" class="Bool"("DisabledEnum"=w377) -> ()  [unwired: 2 in, 2 out]
            n146 = property on="Mover motor" class="Bool"(error in=w378, "DisabledEnum"=w377) -> (error out=w375:errorcluster)  [unwired: 1 in, 1 out]
            n147 = call "Configure trigger.vi"("error in"=w375, "Trigger config"=T10 {"Trigger Source"=1, "Trigger Mode"=0, "Trigger Slope"=0, "Trigger Coupling"=1, "Trigger Level"=0.0}, "Module ID"=w372) -> ("error out"=w374:errorcluster)  [unwired: 8 in]
            n148 = property on="Connect" class="Bool"("DisabledEnum"=T9."Disabled and Grayed Out" ("Disabled")) -> ()  [unwired: 2 in, 2 out]
          }
        }
      }
      frame "Exit" {
        w382 = -1073807346  # Driver was not connected.
        w379 = FALSE ("DAQ lista")
        w394 = Example_States."Wait"  # Not used
        w397 = TRUE  # stop
        # "Se manda paro al motor."
        # "Desconexión del osciloscopio."
        # "Detener tareas de la DAQ."
        # "En el evento Exit se desconectan los equipos y se detiene el motor."
        n149 = Unbundle By Name(w393) -> ("Driver de motor"=w388:refnum<visa-resource-name>, "TDS ID"=w391:i32, "DAQ ID"=w392:i32)
        n150 = property on="DAQ lista" class="Bool (strict)"(error in=w386, "Value"=w379) -> (error out=w387:errorcluster)  [unwired: 1 in, 1 out]
        n151 = property on="Osciloscopio listo" class="Bool (strict)"(error in=w387, "Value"=w379) -> (error out=w381:errorcluster)  [unwired: 1 in, 1 out]
        n152 = property on="Driver listo" class="Bool (strict)"(error in=w381, "Value"=w379) -> (error out=w380:errorcluster)  [unwired: 1 in, 1 out]
        n153 = call "Stop task.vi"("error in"=w380, "Task list"=T11."All", "Module ID"=w392) -> ("error out"=w396:errorcluster)  [unwired: 8 in]
        n154 = call "Disconnect.vi"("error in"=w396, "Module ID"=w391) -> ("error out"=w390:errorcluster)  [unwired: 9 in]
        n155 = call "Stop.vi"("error in (no error)"=w390, "VISA resource name"=w388) -> ("error out"=w389:errorcluster)  [unwired: 8 in, 1 out]
        n156 = call <vilib>:"Clear Errors.vi"("error in (no error)"=w389, "specific error code to clear (0: all)"=w382) -> ("error out"=w383:errorcluster)  [unwired: 4 in, 1 out]
      }
      frame "Error" {
        n157 = case shown="Error 403683" w402 {
          selector: w402 -> [w406 w409 w413]
          tunnel: [w406 w411 w412] -> w401
          frame No Error {
          }
          frame Default {
            n158 = Unbundle By Name(w409) -> ("code"=w408:i32)
            n159 = Format Into String(format string="Error desconocido. Código de error %d.", w408) -> (resulting string=w407:string)  [unwired: 2 in, 1 out]
            n160 = call <vilib>:"Clear Errors.vi"("error in (no error)"=w409) -> ("error out"=w411:errorcluster)  [unwired: 5 in, 1 out]
            n161 = One Button Dialog(message=w407) -> ()  [unwired: 1 in, 1 out]
          }
          frame Error {
            n162 = call <vilib>:"Clear Errors.vi"("error in (no error)"=w413) -> ("error out"=w412:errorcluster)  [unwired: 5 in, 1 out]
            n163 = One Button Dialog(message="No se pudo inicializar uno de los módulos DQMH." ("format string")) -> ()  [unwired: 1 in, 1 out]
          }
        }
      }
    }
    n164 = Select(t=Example_States."Exit", s=w42, f=w44) -> (s? t:f=w43:T8)
  }
  n165 = Unbundle By Name(w11) -> ("DAQ ID"=w6:i32, "TDS ID"=w7:i32, "Driver de motor"=w8:refnum<visa-resource-name>)
  n166 = call "Close.vi"("error in (no error)"=w9, "VISA resource name"=w8) -> ("error out"=w10:errorcluster)  [unwired: 9 in]
  n167 = call "Stop Module.vi"("error in"=w10, "Module ID"=w7) -> ("error out"=w20:errorcluster)  [unwired: 9 in]
  n168 = call "Stop Module.vi"("error in"=w20, "Module ID"=w6) -> ("error out"=w18:errorcluster)  [unwired: 9 in]
  n169 = Unregister For Events(event registration refnum=w17, error in=w18) -> (error out=w16:errorcluster)
  n170 = disable-structure shown="Default" {
    disable-tunnel: w16 -> [w415 _]
    frame condition #0 (active) {
      n171 = call <vilib>:"Simple Error Handler.vi"("error in (no error)"=w415) -> ()  [unwired: 4 in, 5 out]
    }
    frame condition #1 {
      n172 = Quit LabVIEW() -> ()  [unwired: 1 in]
    }
  }
